vi "条形码扫描.vi"() -> ()   [LabVIEW 2014]
panel:
  out "扫描枪显示框":string
  in  "停止":bool
  in  "扫描枪输入框":string
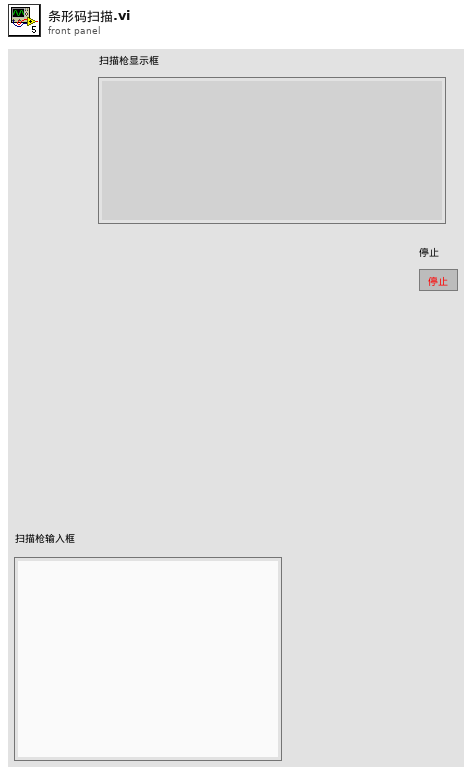
[diagram p1: front panel]
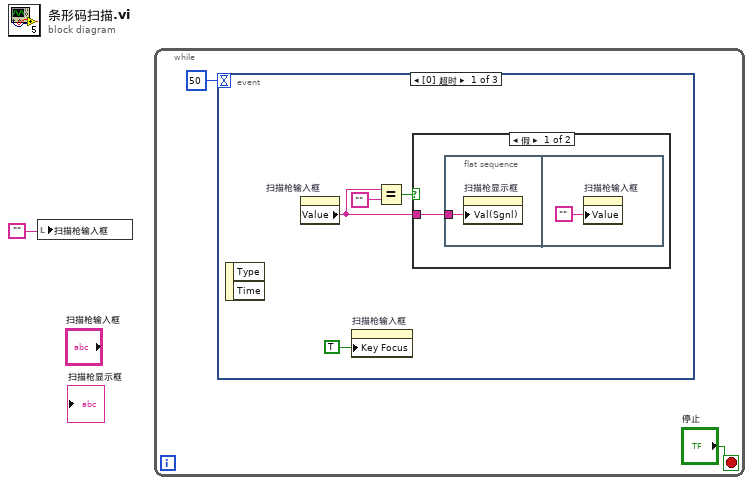
[diagram p0: block diagram]
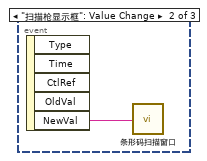
[diagram p3: hidden frame]
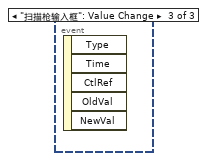
[diagram p4: hidden frame]
diagram:
  n1 = local write "扫描枪输入框"("") -> ()
  n2 = while {
    stop <- "停止" stop-if-true
    n3 = event shown="[0] 超时" {
      selector: _ -> [_ _ _]
      dyn-events: _ -> [_ _ _]
      timeout: 50 -> [_ _ _]
      event Timeout {
        n4 = event-data() -> ()  [unwired: 1 in, 2 out]
        n5 = property on="扫描枪输入框" class="Str"() -> ("Value"=w5:string)  [unwired: 2 in, 2 out]
        n6 = property on="扫描枪输入框" class="Str"("Key Focus"=TRUE ("键选中")) -> ()  [unwired: 2 in, 2 out]
        n7 = Equal?(x=w5, y="") -> (x = y?=w4:bool)
        n8 = case shown="假" w4 {
          tunnel: w5 -> [w8 _]
          frame False {
            n9 = flat-sequence {
              tunnel: w8 -> [w9]
              frame #0 {
                n10 = property on="扫描枪显示框" class="Str"("Val(Sgnl)"=w9) -> ()  [unwired: 2 in, 2 out]
              }
              frame #1 {
                n11 = property on="扫描枪输入框" class="Str"("Value"="") -> ()  [unwired: 2 in, 2 out]
              }
            }
          }
          frame True {
          }
        }
      }
      event "扫描枪显示框": Value Change {
        n12 = event-data() -> ("NewVal"=w11:string)  [unwired: 1 in, 4 out]
        n13 = call "条形码扫描窗口.vi"("扫描的ID号"=w11) -> ()  [unwired: 1 out]
      }
      event "扫描枪输入框": Value Change {
        n14 = event-data() -> ()  [unwired: 1 in, 5 out]
      }
    }
  }
